vi "Network-Discovery Beacon.vi"(0 "name":string, 1 "kill thread notifier":refnum<notifier>, 5 "tcpAddress":string, 7 "tcpPort":u16, 9 "discoveryPort":u16=10001, 11 "interval (ms)":u16=2000) -> ()   [LabVIEW 2020]
uses:
  Typedefs/Network-Server Beacon.ctl
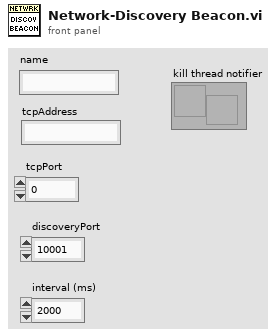
[diagram p1: front panel]
types:
  T1 = typedef "Network-Server Beacon.ctl" = cluster{"name":string, "addr":string, "port":u16, "ver":u16}
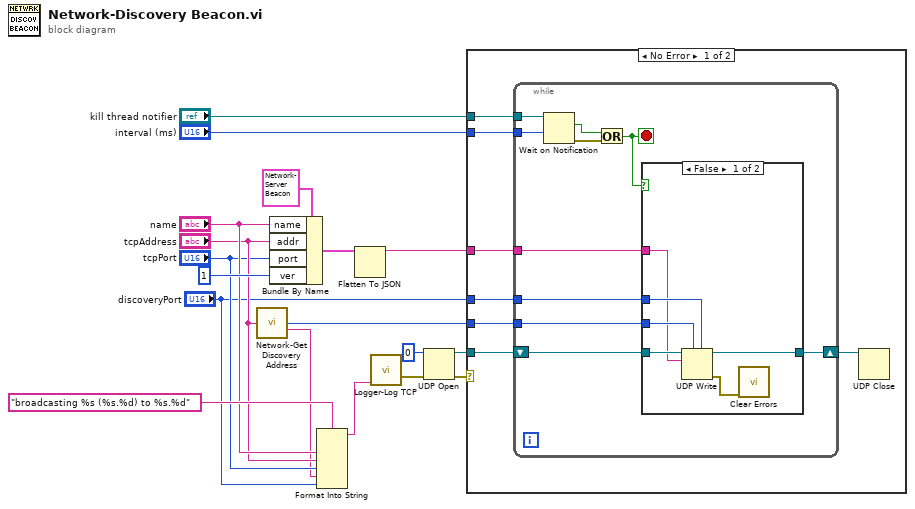
[diagram p0: block diagram]
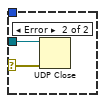
[diagram p3: hidden frame]
diagram:
  n1 = call "Network-Get Discovery Address.vi"("Address"="tcpAddress") -> (8:"subnet address"=w10:u32, 10:"subnet address"=w2:string)  [unwired: 13 in]
  n2 = Bundle By Name(cluster=T1 {"name"="", "addr"="192.168.1.98", "port"=57469, "ver"=10001} ("DiscoveryBeacon"), "name"="name", "addr"="tcpAddress", "port"="tcpPort", "ver"=u16 1 ("Version")) -> (w16:T1)
  n3 = Format Into String(format string="broadcasting %s (%s.%d) to %s.%d", "name", "tcpAddress", "tcpPort", w2, "discoveryPort") -> (resulting string=w1:string)  [unwired: 2 in, 1 out]
  n4 = Flatten To JSON(anything=w16) -> (JSON string=w9:string)  [unwired: 2 in, 1 out]
  n5 = call "Logger-Log TCP.vi"("Message"=w1) -> ("error out"=w8:errorcluster)  [unwired: 14 in]
  n6 = UDP Open(8:w8, 11:0) -> (port=w12:refnum<k16>, 0:w11:errorcluster)  [unwired: 3 in, 1 out]
  n7 = case shown="No Error" w11 {
    selector: w11 -> [_ w44]
    tunnel: "kill thread notifier" -> [w25 _]
    tunnel: "interval (ms)" -> [w24 _]
    tunnel: w9 -> [w23 _]
    tunnel: w12 -> [w22 w43]
    tunnel: w10 -> [w21 _]
    tunnel: "discoveryPort" -> [w20 _]
    frame No Error {
      n8 = while {
        tunnel: w25 -> [w35]
        tunnel: w24 -> [w34]
        tunnel: w23 -> [w31]
        shift-right: [w27] -> w19
        shift-left: w22 -> [w30]
        tunnel: w21 -> [w29]
        tunnel: w20 -> [w28]
        stop <- w26 stop-if-true
        n9 = Wait on Notification(notifier=w35, timeout in ms (-1)=w34) -> (notification=w33:bool, error out=w32:errorcluster)  [unwired: 2 in, 2 out]
        n10 = Or(x=w33, y=w32) -> (x .or. y?=w26:bool)
        n11 = case shown="False" w26 {
          tunnel: w31 -> [w38 _]
          tunnel: w30 -> [w41 w42]
          tunnel: w29 -> [w40 _]
          tunnel: w28 -> [w39 _]
          tunnel: [w37 w42] -> w27
          frame False {
            n12 = UDP Write(address=w40, port or service name=w39, connection ID=w41, data in=w38) -> (error out=w36:errorcluster, 3:w37:refnum<k16>)  [unwired: 2 in]
            n13 = call <vilib>:"Clear Errors.vi"("error in (no error)"=w36) -> ()  [unwired: 5 in, 2 out]
          }
          frame True {
          }
        }
      }
      n14 = UDP Close(connection ID=w19) -> ()  [unwired: 1 in, 2 out]
    }
    frame Error {
      n15 = UDP Close(connection ID=w43, 8:w44) -> ()  [unwired: 2 out]
    }
  }
